vi "DAQ_Micro_Labview.vi"() -> ()   [LabVIEW 2020]
uses:
  <vilib>/Instr/_visa.llb/VISA Configure Serial Port (Instr).vi
panel:
  out "read buffer":string
  in  "Numeric":dbl
  in  "stop":bool
  in  "VISA resource name":refnum<visa-resource-name>
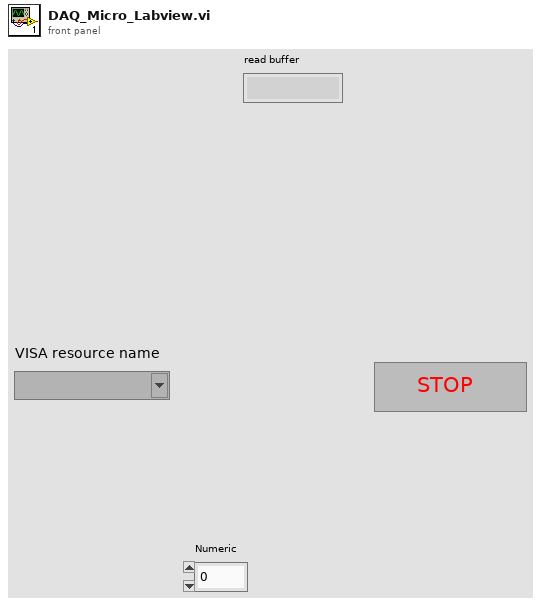
[diagram p1: front panel]
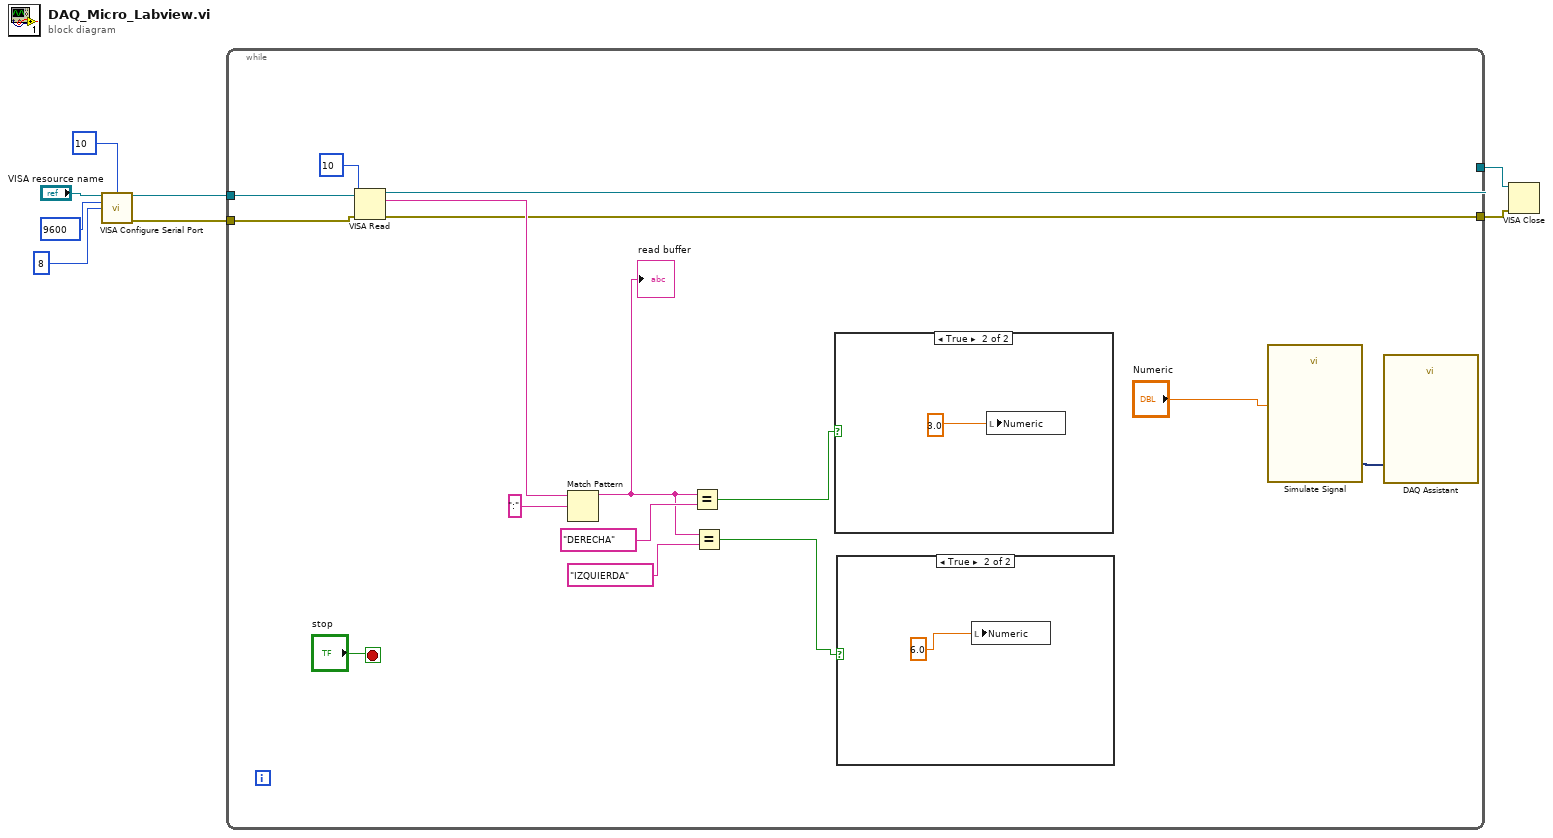
[diagram p0: block diagram]
diagram:
  n1 = call-poly "VISA Configure Serial Port"("VISA resource name"="VISA resource name", "termination char\n(0xA = '\\n' = LF)"=u8 10 ("termination char\n(0xA = '\\n' = LF)"), "baud rate (9600)"=u32 9600, "data bits (8)"=u16 8) -> ("VISA resource name out"=w8:refnum<visa-resource-name>, "error out"=w3:errorcluster)  [unwired: 10 in]
  n2 = while {
    tunnel: w8 -> [w20]
    tunnel: w3 -> [w19]
    tunnel: [w11] -> w2
    tunnel: [w10] -> w1
    stop <- "stop" stop-if-true
    n3 = VISA Read(VISA resource name=w20, byte count=u32 10, error in (no error)=w19) -> (VISA resource name out=w11:refnum<visa-resource-name>, read buffer=w18:string, error out=w10:errorcluster)  [unwired: 1 out]
    n4 = Match Pattern(string=w18, regular expression=":") -> (before substring=w9:string)  [unwired: 1 in, 3 out]
    "read buffer" <- w9
    n5 = Equal?(x=w9, y="DERECHA") -> (x = y?=w15:bool)
    n6 = Equal?(x=w9, y="IZQUIERDA") -> (x = y?=w14:bool)
    n7 = case shown="True" w15 {
      frame False {
      }
      frame True {
        n8 = local write "Numeric"(3.0) -> ()
      }
    }
    n9 = case shown="True" w14 {
      frame False {
      }
      frame True {
        n10 = local write "Numeric"(6.0) -> ()
      }
    }
    n11 = call "Simulate Signal"("Duty Cycle (%)"="Numeric") -> ("Square"=w13:dynamicdata)  [unwired: 13 in, 1 out]
    n12 = call "DAQ Assistant"("data"=w13) -> ()  [unwired: 17 in, 2 out]
  }
  n13 = VISA Close(VISA resource name=w2, error in (no error)=w1) -> ()  [unwired: 1 out]
